vi "Write LiDAR Settings.vi"(8 "error in (no error)":errorcluster, 10 "LiDAR":T1, 11 "LiDAR in":refnum<class "LiDAR.lvclass">) -> (0 "error out":errorcluster, 3 "LiDAR out":refnum<class "LiDAR.lvclass">)   [LabVIEW 2018, in "LiDAR.lvlib" / "LiDAR.lvclass"]
uses:
  LiDAR.lvclass
  PPLs/Configuration/Configuration.lvlibp/Configuration.lvclass
  LiDAR.lvclass/LiDAR.ctl
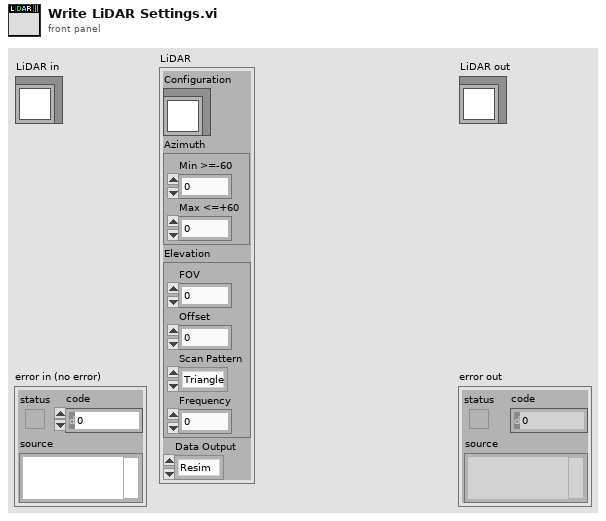
[diagram p1: front panel]
types:
  T1 = cluster{"Configuration":refnum<class "Configuration.lvclass">, "Azimuth":cluster{"Min >=-60":dbl, "Max <=+60 ":dbl}, "Elevation":cluster{"FOV":dbl, "Offset":dbl, "Scan Pattern":enum16{"Triangle", "Snap"}, "Frequency":dbl}, "Data Output":enum16{"Resim", "Point Cloud"}}
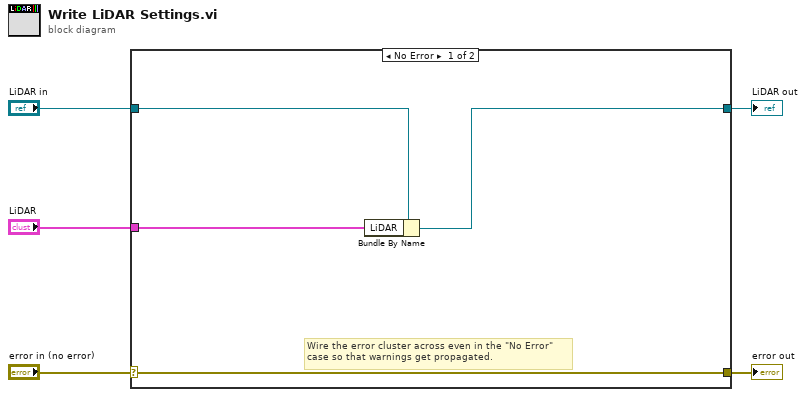
[diagram p0: block diagram]
diagram:
  n1 = case shown="No Error" "error in (no error)" {
    selector: "error in (no error)" -> [w9 w11]
    tunnel: [w9 w11] -> w4
    tunnel: [w6 w10] -> w2
    tunnel: "LiDAR in" -> [w8 w10]
    tunnel: "LiDAR" -> [w7 _]
    frame No Error {
      # "Wire the error cluster across even in the \"No Error\"\ncase so that warnings get propagated."
      n2 = Bundle By Name(cluster=w8, "LiDAR"=w7) -> (w6:refnum<class "LiDAR.lvclass">)
    }
    frame Error {
    }
  }
  "error out" <- w4
  "LiDAR out" <- w2
